vi "Trace at Right Angles.vi"(10 "Start Vectors":T1, 11 "Map in":refnum<class "Maze.lvclass">) -> (3 "Map out":refnum<class "Maze.lvclass">)   [LabVIEW 2021, in "Maze.lvclass"]
uses:
  Maze.lvclass
  Position.ctl
  Maze.lvclass/Maze.ctl
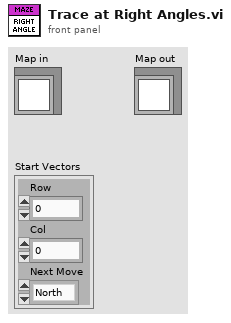
[diagram p1: front panel]
types:
  T1 = typedef "Maze.lvclass/Position.ctl" = cluster{"Row":u64, "Col":u64, "Next Move":enum16{"North", "East", "South", "West", "Halt"}}
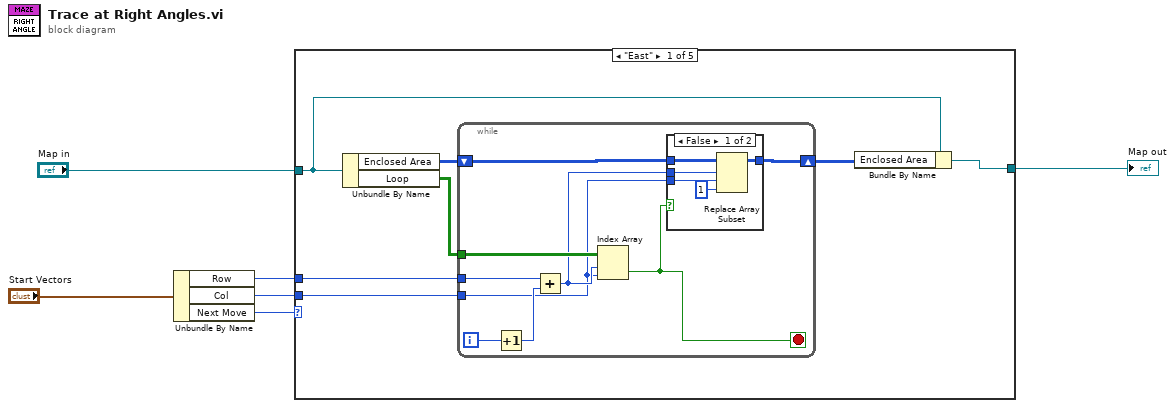
[diagram p0: block diagram]
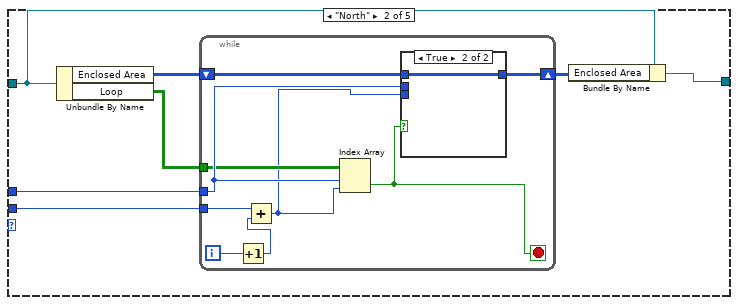
[diagram p3: hidden frame]
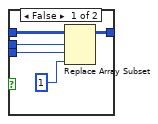
[diagram p4: hidden frame]
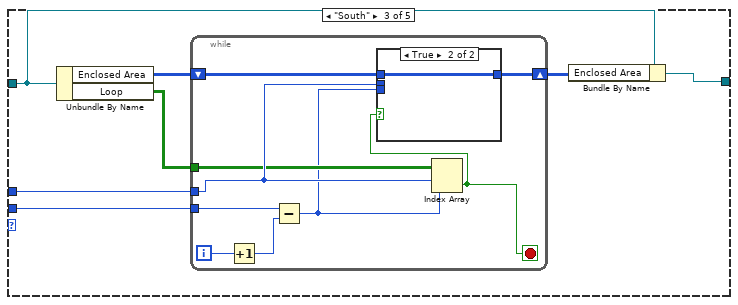
[diagram p5: hidden frame]
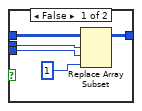
[diagram p6: hidden frame]
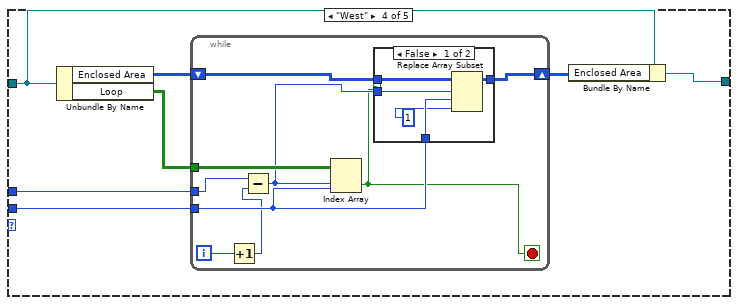
[diagram p7: hidden frame]
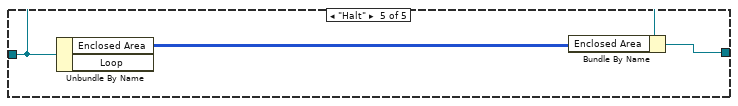
[diagram p9: hidden frame]
diagram:
  n1 = Unbundle By Name("Start Vectors") -> ("Row"=w5:u64, "Col"=w6:u64, "Next Move"=w4:enum16{"North", "East", "South", "West", "Halt"})
  n2 = case shown="\"East\"" w4 {
    tunnel: [w13 w35 w57 w79 w97] -> w2
    tunnel: "Map in" -> [w12 w34 w56 w78 w96]
    tunnel: w5 -> [w11 w33 w55 w77 _]
    tunnel: w6 -> [w9 w31 w53 w75 _]
    frame "East" {
      n3 = Unbundle By Name(w12) -> ("Enclosed Area"=w8:i32[][], "Loop"=w10:bool[][])
      n4 = while {
        tunnel: w11 -> [w22]
        tunnel: w10 -> [w19]
        tunnel: w9 -> [w16]
        shift-right: [w15] -> w7
        shift-left: w8 -> [w18]
        i -> [w21]
        stop <- w14 stop-if-true
        n5 = Increment(x=w21) -> (x+1=w20:i32)
        n6 = Add(x=w22, y=w20) -> (x+y=w17:u64)
        n7 = Index Array(array=w19, index (row)=w17, index (col)=w16) -> (element=w14:bool)
        n8 = case shown="False" w14 {
          tunnel: w18 -> [w27 w28]
          tunnel: w17 -> [w26 _]
          tunnel: w16 -> [w25 _]
          tunnel: [w24 w28] -> w15
          frame False {
            n9 = Replace Array Subset(array=w27, new element=1 ("new element/subarray"), index (row)=w26, index (col)=w25) -> (w24:i32[][])
          }
          frame True {
          }
        }
      }
      n10 = Bundle By Name(cluster=w12, "Enclosed Area"=w7) -> (w13:refnum<class "Maze.lvclass">)
    }
    frame "North" {
      n11 = Unbundle By Name(w34) -> ("Enclosed Area"=w30:i32[][], "Loop"=w32:bool[][])
      n12 = while {
        tunnel: w33 -> [w44]
        tunnel: w32 -> [w42]
        tunnel: w31 -> [w40]
        shift-right: [w39] -> w29
        shift-left: w30 -> [w41]
        i -> [w43]
        stop <- w36 stop-if-true
        n13 = Increment(x=w43) -> (x+1=w37:i32)
        n14 = Add(x=w40, y=w37) -> (x+y=w38:u64)
        n15 = Index Array(array=w42, index (row)=w44, index (col)=w38) -> (element=w36:bool)
        n16 = case shown="True" w36 {
          tunnel: w44 -> [w49 _]
          tunnel: w41 -> [w48 w50]
          tunnel: [w47 w50] -> w39
          tunnel: w38 -> [w45 _]
          frame False {
            n17 = Replace Array Subset(array=w48, new element=1 ("new element/subarray"), index (row)=w49, index (col)=w45) -> (w47:i32[][])
          }
          frame True {
          }
        }
      }
      n18 = Bundle By Name(cluster=w34, "Enclosed Area"=w29) -> (w35:refnum<class "Maze.lvclass">)
    }
    frame "South" {
      n19 = Unbundle By Name(w56) -> ("Enclosed Area"=w52:i32[][], "Loop"=w54:bool[][])
      n20 = while {
        tunnel: w55 -> [w66]
        tunnel: w54 -> [w64]
        tunnel: w53 -> [w62]
        shift-right: [w61] -> w51
        shift-left: w52 -> [w63]
        i -> [w65]
        stop <- w58 stop-if-true
        n21 = Increment(x=w65) -> (x+1=w59:i32)
        n22 = Subtract(x=w62, y=w59) -> (x-y=w60:u64)
        n23 = Index Array(array=w64, index (row)=w66, index (col)=w60) -> (element=w58:bool)
        n24 = case shown="True" w58 {
          tunnel: w66 -> [w71 _]
          tunnel: w63 -> [w70 w72]
          tunnel: [w69 w72] -> w61
          tunnel: w60 -> [w67 _]
          frame False {
            n25 = Replace Array Subset(array=w70, new element=1 ("new element/subarray"), index (row)=w71, index (col)=w67) -> (w69:i32[][])
          }
          frame True {
          }
        }
      }
      n26 = Bundle By Name(cluster=w56, "Enclosed Area"=w51) -> (w57:refnum<class "Maze.lvclass">)
    }
    frame "West" {
      n27 = Unbundle By Name(w78) -> ("Enclosed Area"=w74:i32[][], "Loop"=w76:bool[][])
      n28 = while {
        tunnel: w77 -> [w88]
        tunnel: w76 -> [w86]
        tunnel: w75 -> [w84]
        shift-right: [w83] -> w73
        shift-left: w74 -> [w85]
        i -> [w87]
        stop <- w80 stop-if-true
        n29 = Increment(x=w87) -> (x+1=w81:i32)
        n30 = Subtract(x=w88, y=w81) -> (x-y=w82:u64)
        n31 = Index Array(array=w86, index (row)=w82, index (col)=w84) -> (element=w80:bool)
        n32 = case shown="False" w80 {
          tunnel: w85 -> [w93 w94]
          tunnel: w84 -> [w92 _]
          tunnel: [w91 w94] -> w83
          tunnel: w82 -> [w89 _]
          frame False {
            n33 = Replace Array Subset(array=w93, new element=1 ("new element/subarray"), index (row)=w89, index (col)=w92) -> (w91:i32[][])
          }
          frame True {
          }
        }
      }
      n34 = Bundle By Name(cluster=w78, "Enclosed Area"=w73) -> (w79:refnum<class "Maze.lvclass">)
    }
    frame "Halt" {
      n35 = Unbundle By Name(w96) -> ("Enclosed Area"=w95:i32[][])  [unwired: 1 out]
      n36 = Bundle By Name(cluster=w96, "Enclosed Area"=w95) -> (w97:refnum<class "Maze.lvclass">)
    }
  }
  "Map out" <- w2
